vi "Find drivers DLL.vi"(8 "error in (no error)":errorcluster, 10 "Path to LUT":path=path "C:/Program Files (x86)/National Instruments/LabVIEW 2017/instr.lib/ANC350/ANRv51-C4-124.LUT", 11 "Path to DLL":path=path "C:/Program Files (x86)/National Instruments/LabVIEW 2017/instr.lib/ANC350/Win64/anc350v4.dll") -> (0 "error out":errorcluster, 2 "LUT path out":path=path "C:/Program Files (x86)/National Instruments/LabVIEW 2017/instr.lib/ANC350/Win64/anc350v4.dll", 3 "path out":path=path "C:/Program Files (x86)/National Instruments/LabVIEW 2017/instr.lib/ANC350/Win64/anc350v4.dll")   [LabVIEW 2022 SP3, in "SampleRotator.lvlib"]
doc: "At first, verifies given path. If the path is incorrect, searches in library directory, and in \"LabVIEW/instr directory\". If cannot find the driver DLL, it will prompt an user.\n\ninputs: path.\n\nOutputs: path; error cluster."
uses:
  SampleRotator.lvlib
  <vilib>/Utility/sysdir.llb/System Directory Type.ctl
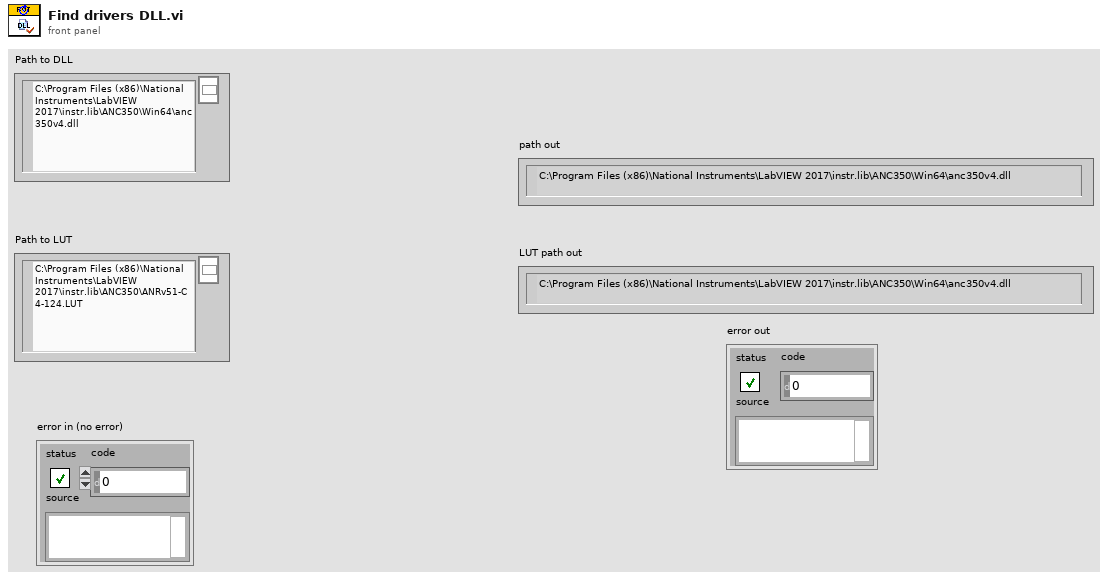
[diagram p1: front panel]
types:
  T1 = typedef "System Directory Type.ctl" = i32
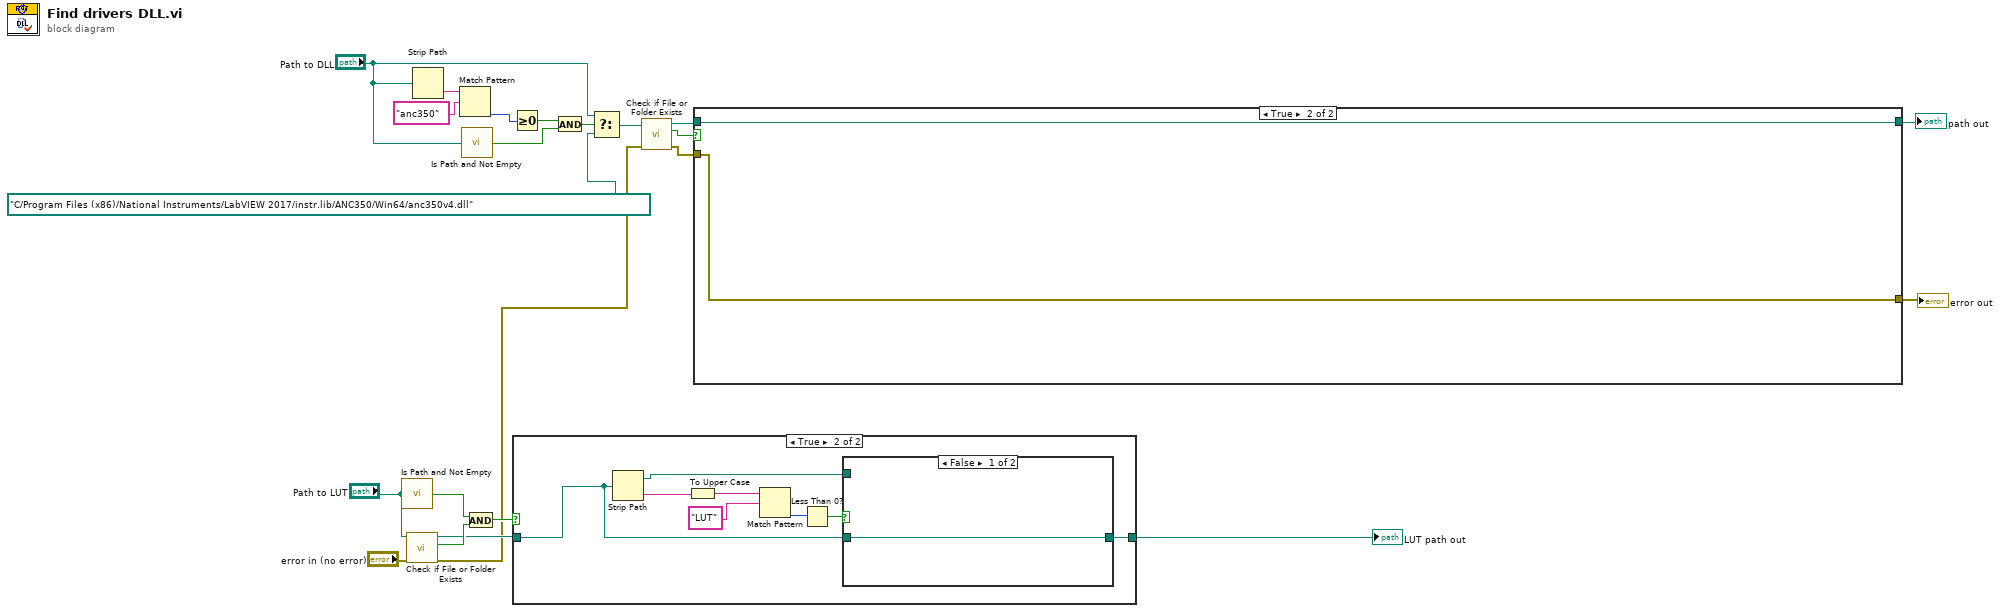
[diagram p0: block diagram]
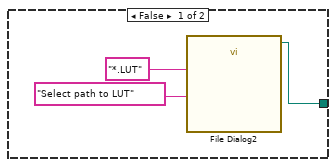
[diagram p2: hidden frame]
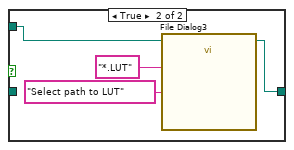
[diagram p3: hidden frame]
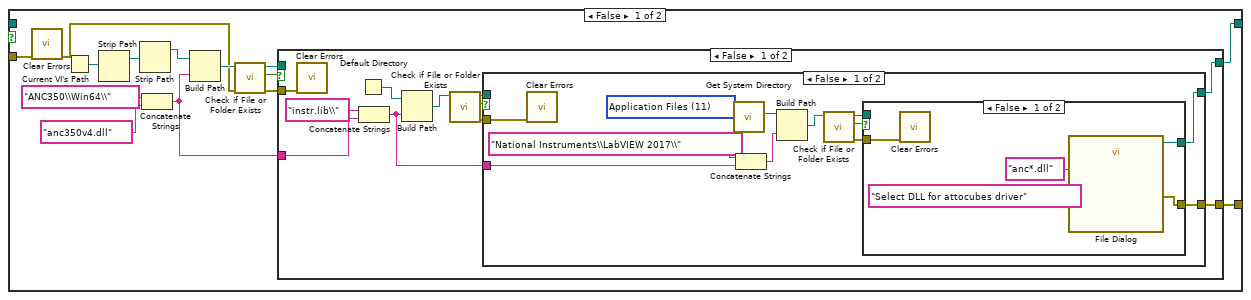
[diagram p4: hidden frame]
diagram:
  n1 = call <vilib>:"Is Path and Not Empty.vi"("path"="Path to LUT") -> ("Is Path and Not Empty?"=w7:bool)  [unwired: 4 in]
  n2 = call <vilib>:"Check if File or Folder Exists.vi"("error in (no error)"="error in (no error)", "path"="Path to LUT") -> ("error out"=w2:errorcluster, "file or folder exists?"=w6:bool, "dup path"=w4:path)  [unwired: 7 in]
  n3 = Strip Path(path="Path to DLL") -> (name=w15:string)  [unwired: 1 out]
  n4 = Match Pattern(string=w15, regular expression="anc350" ("pattern (all files)")) -> (offset past match=w13:i32)  [unwired: 1 in, 3 out]
  n5 = call <vilib>:"Is Path and Not Empty.vi"("path"="Path to DLL") -> ("Is Path and Not Empty?"=w9:bool)  [unwired: 4 in]
  n6 = And(x=w7, y=w6) -> (x .and. y?=w5:bool)
  n7 = Greater Or Equal To 0?(x=w13) -> (x >= 0?=w11:bool)
  n8 = case shown="True" w5 {
    tunnel: w4 -> [_ w26]
    tunnel: [w23 w29] -> w3
    frame False {
      n9 = call "File Dialog2"("prompt"="Select path to LUT", "pattern (all files)"="*.LUT") -> ("selected path"=w23:path)  [unwired: 10 in, 3 out]
    }
    frame True {
      n10 = Strip Path(path=w26) -> (stripped path=w28:path, name=w33:string)
      n11 = To Upper Case(1:w33) -> (0:w32:string)
      n12 = Match Pattern(string=w32, regular expression="LUT") -> (offset past match=w30:i32)  [unwired: 1 in, 3 out]
      n13 = Less Than 0?(x=w30) -> (x < 0?=w27:bool)
      n14 = case shown="False" w27 {
        tunnel: [w34 w36] -> w29
        tunnel: w28 -> [_ w35]
        tunnel: w26 -> [w34 _]
        frame False {
        }
        frame True {
          n15 = call "File Dialog3"("start path"=w35, "prompt"="Select path to LUT", "pattern (all files)"="*.LUT") -> ("selected path"=w36:path)  [unwired: 9 in, 3 out]
        }
      }
    }
  }
  "LUT path out" <- w3
  n16 = And(x=w11, y=w9) -> (x .and. y?=w12:bool)
  n17 = Select(t="Path to DLL", s=w12, f=path "C:/Program Files (x86)/National Instruments/LabVIEW 2017/instr.lib/ANC350/Win64/anc350v4.dll" ("Path to *.DLL 2")) -> (s? t:f=w19:path)
  n18 = call <vilib>:"Check if File or Folder Exists.vi"("error in (no error)"=w2, "path"=w19) -> ("error out"=w20:errorcluster, "file or folder exists?"=w18:bool, "dup path"=w17:path)  [unwired: 7 in]
  n19 = case shown="True" w18 {
    tunnel: w17 -> [_ w88]
    tunnel: [w43 w88] -> w22
    tunnel: [w42 w87] -> w21
    tunnel: w20 -> [w40 w87]
    frame False {
      n20 = call <vilib>:"Clear Errors.vi"("error in (no error)"=w40) -> ("error out"=w39:errorcluster)  [unwired: 5 in, 1 out]
      n21 = Current VI's Path() -> (path=w52:path)
      n22 = Strip Path(path=w52) -> (stripped path=w51:path)  [unwired: 1 out]
      n23 = Strip Path(path=w51) -> (stripped path=w50:path)  [unwired: 1 out]
      n24 = Concatenate Strings("ANC350\\Win64\\" ("name or relative path"), "anc350v4.dll" ("string")) -> (w44:string)
      n25 = Build Path(base path=w50, name or relative path=w44) -> (appended path=w49:path)
      n26 = call <vilib>:"Check if File or Folder Exists.vi"("error in (no error)"=w39, "path"=w49) -> ("error out"=w41:errorcluster, "file or folder exists?"=w46:bool, "dup path"=w45:path)  [unwired: 7 in]
      n27 = case shown="False" w46 {
        tunnel: w45 -> [_ w86]
        tunnel: [w56 w86] -> w43
        tunnel: w44 -> [w61 _]
        tunnel: [w55 w85] -> w42
        tunnel: w41 -> [w53 w85]
        frame False {
          n28 = call <vilib>:"Clear Errors.vi"("error in (no error)"=w53) -> ()  [unwired: 5 in, 2 out]
          n29 = Default Directory() -> (w63:path)
          n30 = Concatenate Strings("instr.lib\\" ("string"), w61) -> (w58:string)
          n31 = Build Path(base path=w63, name or relative path=w58) -> (appended path=w60:path)
          n32 = call <vilib>:"Check if File or Folder Exists.vi"("path"=w60) -> ("error out"=w54:errorcluster, "file or folder exists?"=w59:bool, "dup path"=w57:path)  [unwired: 8 in]
          n33 = case shown="False" w59 {
            tunnel: w58 -> [w71 _]
            tunnel: w57 -> [_ w84]
            tunnel: [w67 w84] -> w56
            tunnel: [w66 w83] -> w55
            tunnel: w54 -> [w64 w83]
            frame False {
              w75 = T1 11 items=["User Home"=0, "User Desktop"=1, "User Documents"=2, "User Application Data"=3, "User Preferences"=4, "User Temporary"=5, "Public Documents"=6, "Public Application Data"=7, "Public Preferences"=8, "Public Cache"=13, "System Core Libraries"=9, "System Installed Libraries"=10, "Application Files"=11, "Boot Volume Root"=12] ("system directory type")
              n34 = call <vilib>:"Clear Errors.vi"("error in (no error)"=w64) -> ()  [unwired: 5 in, 2 out]
              n35 = call <vilib>:"Get System Directory.vi"("system directory type"=w75) -> ("system directory"=w74:path)  [unwired: 10 in]
              n36 = Concatenate Strings("National Instruments\\LabVIEW 2017\\", w71) -> (w72:string)
              n37 = Build Path(base path=w74, name or relative path=w72) -> (appended path=w70:path)
              n38 = call <vilib>:"Check if File or Folder Exists.vi"("path"=w70) -> ("error out"=w65:errorcluster, "file or folder exists?"=w68:bool, "dup path"=w69:path)  [unwired: 8 in]
              n39 = case shown="False" w68 {
                tunnel: w69 -> [_ w82]
                tunnel: [w77 w82] -> w67
                tunnel: [w78 w81] -> w66
                tunnel: w65 -> [w76 w81]
                frame False {
                  n40 = call <vilib>:"Clear Errors.vi"("error in (no error)"=w76) -> ()  [unwired: 5 in, 2 out]
                  n41 = call "File Dialog"("prompt"="Select DLL for attocubes driver", "pattern (all files)"="anc*.dll") -> ("selected path"=w77:path, "error out"=w78:errorcluster)  [unwired: 10 in, 2 out]
                }
                frame True {
                }
              }
            }
            frame True {
            }
          }
        }
        frame True {
        }
      }
    }
    frame True {
    }
  }
  "path out" <- w22
  "error out" <- w21
